vi "Omron Serial FINS-Request And Respond.vi"(8 "error in":errorcluster, 11 "Buffer Data In":T1={"VISA Resource Name"="", "Wait For Read(ms)"=50, "Command Code"=enum."Memory area read", "Command String"="", "Read Bytes"=0, "Response String"=""}) -> (0 "error out":errorcluster, 3 "Buffer Data Out":T1={"VISA Resource Name"="", "Wait For Read(ms)"=50, "Command Code"=enum."Memory area read", "Command String"="", "Read Bytes"=0, "Response String"=""})   [LabVIEW 2016]
uses:
  Data Def/Omron Serial FINS-Buffer Data.ctl
  Data Def/Omron Serial FINS-Command Code.ctl
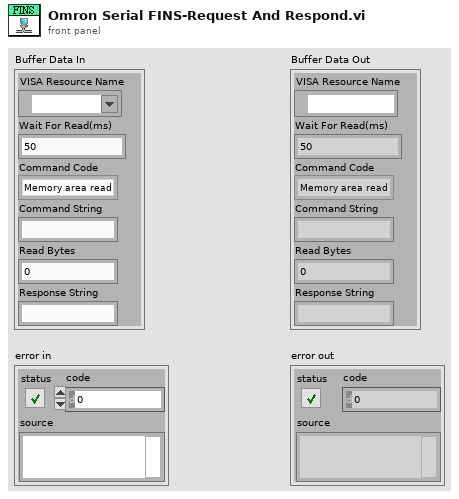
[diagram p1: front panel]
types:
  T1 = typedef "Omron Serial FINS-Buffer Data.ctl" = cluster{"VISA Resource Name":refnum<visa-resource-name>, "Wait For Read(ms)":u32, "Command Code":T2, "Command String":string, "Read Bytes":u32, "Response String":string}
  T2 = typedef "Omron Serial FINS-Command Code.ctl" = enum16{"Memory area read", "Memory area write"}
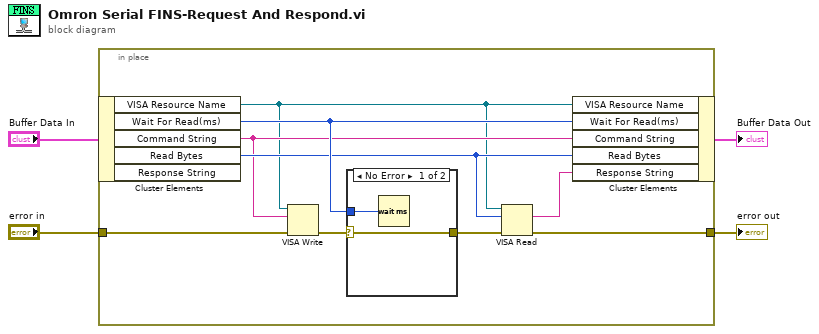
[diagram p0: block diagram]
diagram:
  n1 = in-place {
    in-place-border: "error in" -> [w13]
    in-place-border: [w10] -> w3
    n2 = in-place-cluster #1("Buffer Data In") -> ("VISA Resource Name"=w5:refnum<visa-resource-name>, "Wait For Read(ms)"=w11:u32, "Command String"=w6:string, "Read Bytes"=w8:u32)  [unwired: 1 out]
    n3 = VISA Write(VISA resource name=w5, write buffer=w6, error in (no error)=w13) -> (error out=w12:errorcluster)  [unwired: 2 out]
    n4 = case shown="No Error" w12 {
      selector: w12 -> [w14 w16]
      tunnel: w11 -> [w15 _]
      tunnel: [w14 w16] -> w9
      frame No Error {
        n5 = Wait (ms)(milliseconds to wait=w15) -> ()  [unwired: 1 out]
      }
      frame Error {
      }
    }
    n6 = VISA Read(VISA resource name=w5, byte count=w8, error in (no error)=w9) -> (read buffer=w7:string, error out=w10:errorcluster)  [unwired: 2 out]
    n7 = in-place-cluster #1("VISA Resource Name"=w5, "Wait For Read(ms)"=w11, "Command String"=w6, "Read Bytes"=w8, "Response String"=w7) -> (→"Buffer Data Out":T1)
  }
  "error out" <- w3
